vi "Chroma 1905x Series Configure AC Real Current Limit Query.vi"(6 "Mode":u16(ring) items=["AC"], 7 "error in (no error)":errorcluster, 9 "Step":T1=1 min=1 max=99 step=1, 10 "VISA resource name":refnum<visa-resource-name>) -> (0 "error out":errorcluster, 2 "Current value [A]":string, 3 "VISA resource name out":refnum<visa-resource-name>)   [LabVIEW 2025]
uses:
  Type Def/steps--numeric.ctl
panel:
  # "Real Current Limit query"
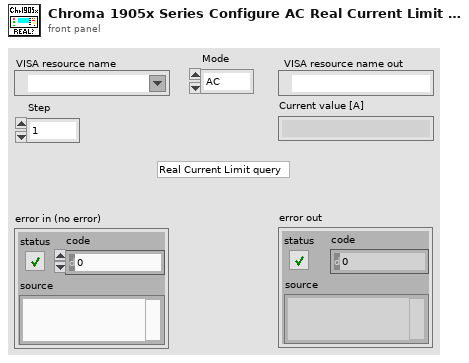
[diagram p1: front panel]
types:
  T1 = typedef "steps--numeric.ctl" = u8
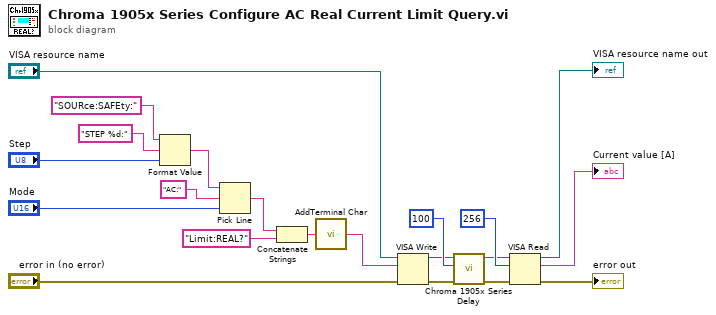
[diagram p0: block diagram]
diagram:
  n1 = Format Value(string ("")="SOURce:SAFEty:", format string="STEP %d:", value (0)="Step") -> (output string=w16:string)
  n2 = Pick Line(string ("")=w16, multi-line string="AC:", line index="Mode") -> (output string=w13:string)
  n3 = Concatenate Strings(w13, "Limit:REAL?" ("format string")) -> (w15:string)
  n4 = call "AddTerminal Char.vi"("Cmd string"=w15) -> ("Concatenated String"=w5:string)  [unwired: 4 in]
  n5 = VISA Write(VISA resource name="VISA resource name", write buffer=w5, error in (no error)="error in (no error)") -> (VISA resource name out=w9:refnum<visa-resource-name>, error out=w7:errorcluster)  [unwired: 1 out]
  n6 = call "Chroma 1905x Series Delay.vi"("error in (no error)"=w7, "Time Delay [ms]"=u32 100 ("Time Delay ms"), "VISA resource name"=w9) -> ("error out"=w8:errorcluster, "VISA resource name 2"=w10:refnum<visa-resource-name>)  [unwired: 7 in]
  n7 = VISA Read(VISA resource name=w10, byte count=u32 256, error in (no error)=w8) -> (VISA resource name out=→"VISA resource name out":refnum<visa-resource-name>, read buffer=→"Current value [A]":string, error out=→"error out":errorcluster)  [unwired: 1 out]
